vi "Set Security Level CORE.vi"(8 "error in (no error)":errorcluster, 9 "Set or Clear":T1, 10 "New Level":T2, 11 "Motion Detector in":refnum<class "Motion Detectors.lvclass">) -> (0 "error out":errorcluster, 2 "Last Action Performed":string, 3 "Motion Detector out":refnum<class "Motion Detectors.lvclass">)   [LabVIEW 2014, in "Motion Detectors.lvclass"]
uses:
  Motion Detectors.lvclass
  Security System/Security Level.ctl
  Security System/Set or Clear.ctl
  Motion Detectors.lvclass/Motion Detectors.ctl
  Motion Mode.ctl
  Security System/Security System.lvclass
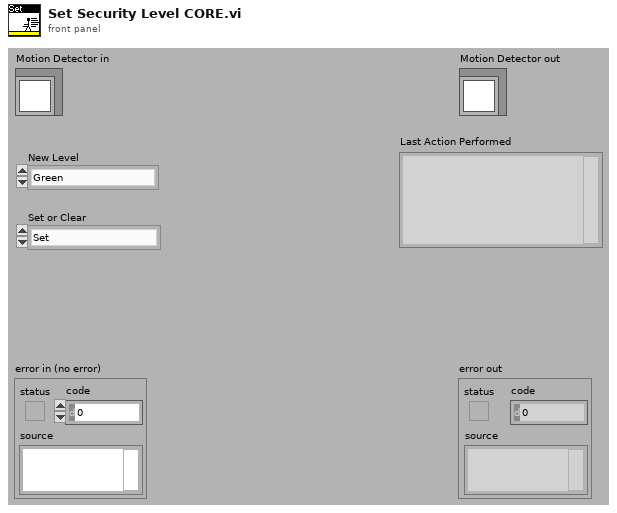
[diagram p1: front panel]
types:
  T1 = typedef "Security System.lvclass/Set or Clear.ctl" = enum16{"Set", "Clear"}
  T2 = typedef "Security System.lvclass/Security Level.ctl" = enum16{"Green", "Yellow", "Orange", "Red"}
  T3 = typedef "Motion Detectors.lvclass/Motion Mode.ctl" = enum16{"Visual Spectrum", "Infrared + Visual", "Infrared + Heat + Visual"}
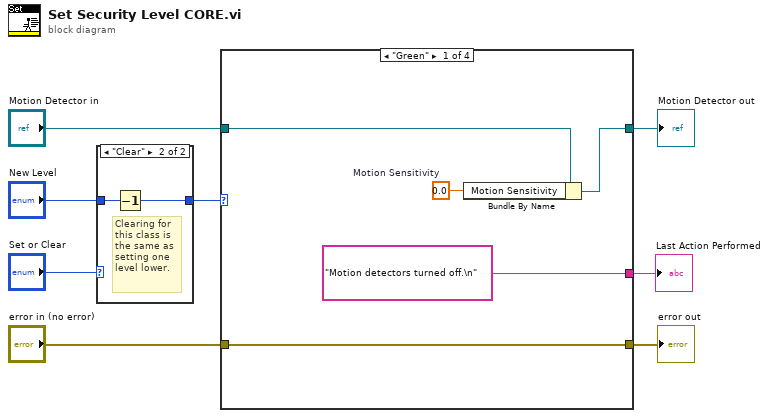
[diagram p0: block diagram]
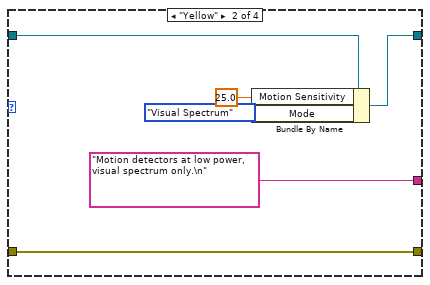
[diagram p3: hidden frame]
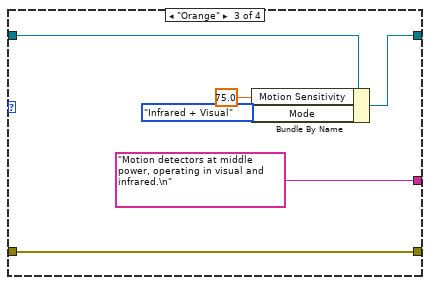
[diagram p4: hidden frame]
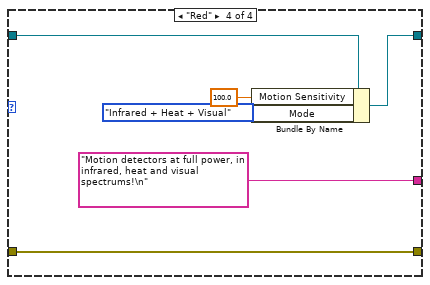
[diagram p5: hidden frame]
diagram:
  n1 = case shown="\"Clear\"" "Set or Clear" {
    tunnel: "New Level" -> [w9 w11]
    tunnel: [w9 w10] -> w2
    frame "Set" {
    }
    frame "Clear" {
      # "Clearing for this class is the same as setting one level lower."
      n2 = Decrement(x=w11) -> (x-1=w10:T2)
    }
  }
  n3 = case shown="\"Green\"" w2 {
    tunnel: [w14 w20 w26 w32] -> w5
    tunnel: "Motion Detector in" -> [w15 w21 w27 w33]
    tunnel: [w16 w22 w28 w34] -> w7
    tunnel: "error in (no error)" -> [w16 w22 w28 w34]
    tunnel: ["Motion detectors turned off.\n" ("Last Action Performed") "Motion detectors at low power, visual spectrum only.\n" ("Last Action Performed") "Motion detectors at middle power, operating in visual and infrared.\n" ("Last Action Performed") "Motion detectors at full power, in infrared, heat and visual spectrums!\n" ("Last Action Performed")] -> w1
    frame "Green" {
      w13 = 0.0  # Motion Sensitivity
      n4 = Bundle By Name(cluster=w15, "Motion Sensitivity"=w13) -> (w14:refnum<class "Motion Detectors.lvclass">)
    }
    frame "Yellow" {
      n5 = Bundle By Name(cluster=w21, "Motion Sensitivity"=25.0, "Mode"=Motion_Mode."Visual Spectrum") -> (w20:refnum<class "Motion Detectors.lvclass">)
    }
    frame "Orange" {
      n6 = Bundle By Name(cluster=w27, "Motion Sensitivity"=75.0, "Mode"=Motion_Mode."Infrared + Visual") -> (w26:refnum<class "Motion Detectors.lvclass">)
    }
    frame "Red" {
      n7 = Bundle By Name(cluster=w33, "Motion Sensitivity"=100.0, "Mode"=Motion_Mode."Infrared + Heat + Visual") -> (w32:refnum<class "Motion Detectors.lvclass">)
    }
  }
  "error out" <- w7
  "Motion Detector out" <- w5
  "Last Action Performed" <- w1
